vi "Table_GetNodeInformation.vi"(8 "error in (no error)":errorcluster, 9 "TreeBrowser":refnum<k24>, 11 "reference":refnum<k24>) -> (0 "error IO":errorcluster, 3 "Channels":T1[](array[typedef]))   [LabVIEW 2012, in "TableSupportLib.lvlib"]
uses:
  TableSupportLib.lvlib
  NationalInstruments.VeriStand.SystemStorage
  Table_ChannelInfoCluster.ctl
  NationalInstruments.VeriStand.SystemStorageUI
  NationalInstruments.VeriStand.SystemDefinitionAPI
  <vilib>/NI Veristand/Custom Device Offline API/Custom Device Offline API.lvlib
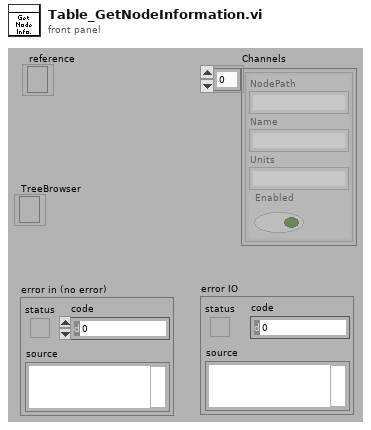
[diagram p1: front panel]
types:
  T1 = typedef "TableSupportLib.lvlib/Table_ChannelInfoCluster.ctl" = cluster{"NodePath":string, "Name":string, "Units":string, "Enabled":bool}
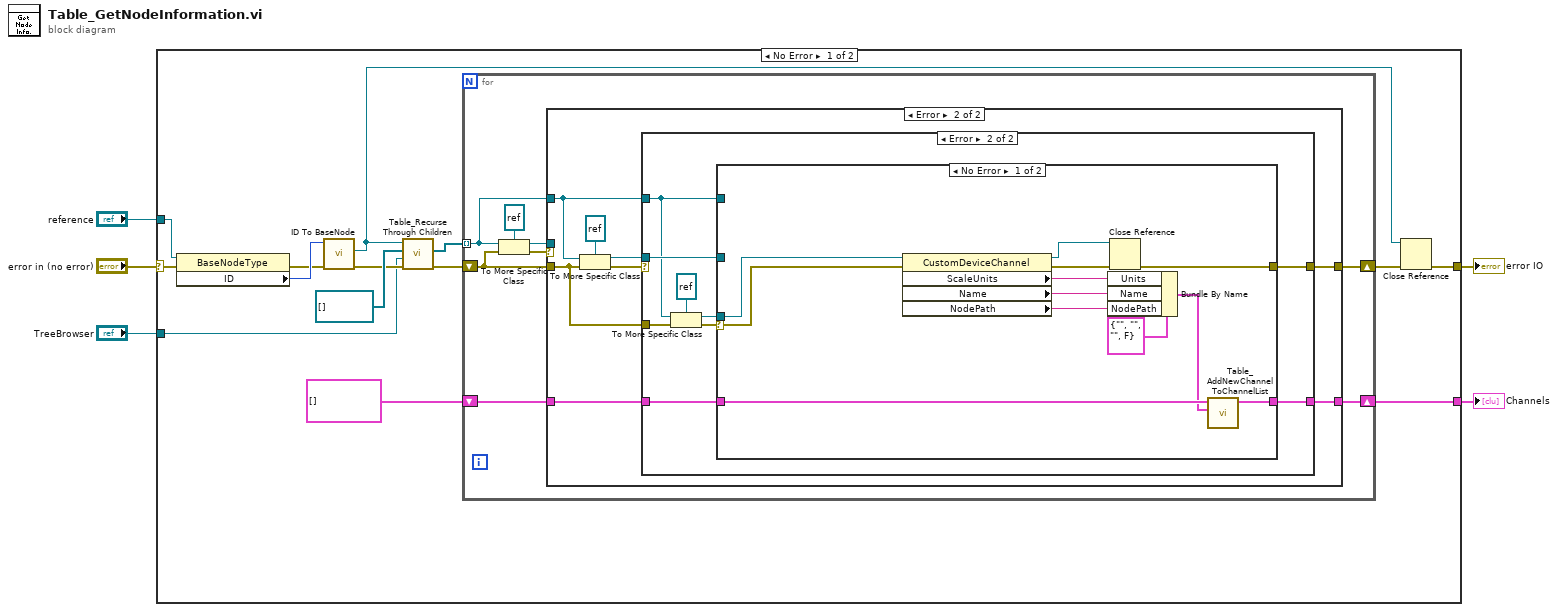
[diagram p0: block diagram]
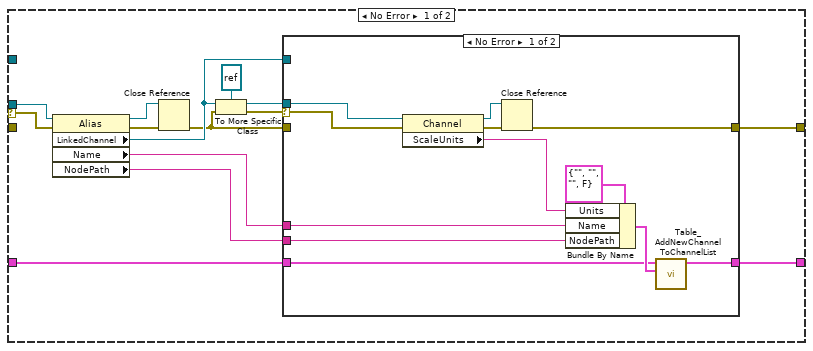
[diagram p2: hidden frame]
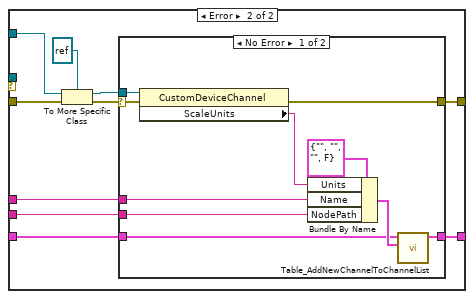
[diagram p3: hidden frame]
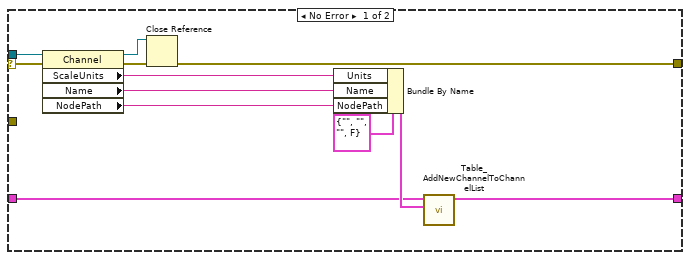
[diagram p5: hidden frame]
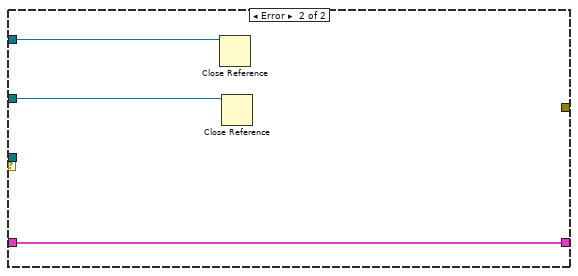
[diagram p6: hidden frame]
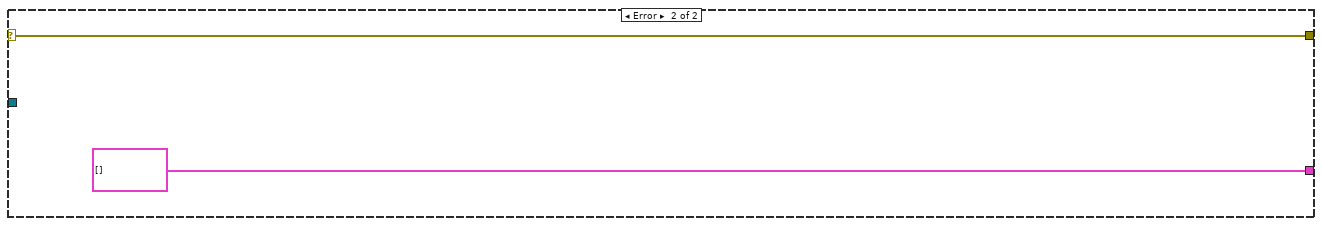
[diagram p7: hidden frame]
diagram:
  n1 = case shown="No Error" "error in (no error)" {
    selector: "error in (no error)" -> [w17 w120]
    tunnel: "reference" -> [w18 _]
    tunnel: [w12 T1[] []] -> w2
    tunnel: [w9 w120] -> w4
    tunnel: "TreeBrowser" -> [w6 _]
    frame No Error {
      n2 = property class="BaseNodeType"(reference=w18, error in=w17) -> (error out=w16:errorcluster, "ID"=w19:u64)  [unwired: 1 out]
      n3 = call <vilib>:"ID To BaseNode.vi"("error in (no error)"=w16, "ID in"=w19) -> ("error out"=w14:errorcluster, "BaseNode"=w7:refnum<k24>)  [unwired: 7 in, 1 out]
      n4 = call "Table_Recurse Through Children.vi"("error in"=w14, "TreeBrowser"=w6, "Children"=refnum<k24>[] [], ".NET Refnum in"=w7) -> ("error out"=w8:errorcluster, "Children"=w11:refnum<k24>[])  [unwired: 6 in]
      n5 = for {
        tunnel: w11 -> [w20] mode=indexing
        shift-right: [w24] -> w12
        shift-left: T1[] [] -> [w23]
        shift-right: [w22] -> w10
        shift-left: w8 -> [w25]
        n6 = To More Specific Class(target class=refnum<k24> refnum ("new reference"), reference=w20, error in=w25) -> (specific class reference=w21:refnum<k24>, error out=w26:errorcluster)
        n7 = case shown="Error" w26 {
          selector: w26 -> [w40 _]
          tunnel: [w34 w82] -> w22
          tunnel: w21 -> [w39 _]
          tunnel: w20 -> [_ w78]
          tunnel: w25 -> [_ w75]
          tunnel: [w35 w77] -> w24
          tunnel: w23 -> [w31 w76]
          frame No Error {
            n8 = property class="Alias"(reference=w39, error in=w40) -> (reference out=w36:refnum<k24>, error out=w37:errorcluster, "LinkedChannel"=w29:refnum<k24>, "Name"=w33:string, "NodePath"=w32:string)
            n9 = Close Reference(reference=w36, error in (no error)=w37) -> (error out=w28:errorcluster)
            n10 = To More Specific Class(target class=refnum<k24> refnum ("new reference"), reference=w29, error in=w28) -> (specific class reference=w38:refnum<k24>, error out=w30:errorcluster)
            n11 = case shown="No Error" w30 {
              selector: w30 -> [w42 _]
              tunnel: w38 -> [w53 _]
              tunnel: [w52 w56] -> w35
              tunnel: [w50 w58] -> w34
              tunnel: w33 -> [w45 w54]
              tunnel: w32 -> [w44 w55]
              tunnel: w31 -> [w43 w57]
              tunnel: w29 -> [_ w63]
              tunnel: w28 -> [_ w62]
              frame No Error {
                n12 = property class="Channel"(reference=w53, error in=w42) -> (reference out=w49:refnum<k24>, error out=w51:errorcluster, "ScaleUnits"=w46:string)
                n13 = Close Reference(reference=w49, error in (no error)=w51) -> (error out=w50:errorcluster)
                n14 = Bundle By Name(cluster=T1 {"NodePath"="", "Name"="", "Units"="", "Enabled"=FALSE}, "Units"=w46, "Name"=w45, "NodePath"=w44) -> (w47:T1)
                n15 = call "Table_AddNewChannelToChannelList.vi"("Channel"=w47, "Channels"=w43) -> ("Channels Out"=w52:T1[])  [unwired: 9 in]
              }
              frame Error {
                n16 = To More Specific Class(target class=refnum<k24> refnum ("new reference"), reference=w63, error in=w62) -> (specific class reference=w60:refnum<k24>, error out=w59:errorcluster)
                n17 = case shown="No Error" w59 {
                  selector: w59 -> [w72 _]
                  tunnel: w60 -> [w73 _]
                  tunnel: [w71 _] -> w58
                  tunnel: w57 -> [w68 w74]
                  tunnel: [w67 w74] -> w56
                  tunnel: w55 -> [w66 _]
                  tunnel: w54 -> [w65 _]
                  frame No Error {
                    n18 = property class="CustomDeviceChannel"(reference=w73, error in=w72) -> (error out=w71:errorcluster, "ScaleUnits"=w64:string)  [unwired: 1 out]
                    n19 = Bundle By Name(cluster=T1 {"NodePath"="", "Name"="", "Units"="", "Enabled"=FALSE}, "Units"=w64, "Name"=w65, "NodePath"=w66) -> (w69:T1)
                    n20 = call "Table_AddNewChannelToChannelList.vi"("Channel"=w69, "Channels"=w68) -> ("Channels Out"=w67:T1[])  [unwired: 9 in]
                  }
                  frame Error {
                  }
                }
              }
            }
          }
          frame Error {
            n21 = To More Specific Class(target class=refnum<k24> refnum ("new reference"), reference=w78, error in=w75) -> (specific class reference=w80:refnum<k24>, error out=w79:errorcluster)
            n22 = case shown="Error" w79 {
              selector: w79 -> [w93 _]
              tunnel: [w90 w95] -> w82
              tunnel: w80 -> [w85 w103]
              tunnel: w78 -> [_ w100]
              tunnel: [w86 w96] -> w77
              tunnel: w76 -> [w87 w97]
              tunnel: w75 -> [_ w101]
              frame No Error {
                n23 = property class="Channel"(reference=w85, error in=w93) -> (reference out=w89:refnum<k24>, error out=w91:errorcluster, "ScaleUnits"=w83:string, "Name"=w94:string, "NodePath"=w84:string)
                n24 = Close Reference(reference=w89, error in (no error)=w91) -> (error out=w90:errorcluster)
                n25 = Bundle By Name(cluster=T1 {"NodePath"="", "Name"="", "Units"="", "Enabled"=FALSE}, "Units"=w83, "Name"=w94, "NodePath"=w84) -> (w88:T1)
                n26 = call "Table_AddNewChannelToChannelList.vi"("Channel"=w88, "Channels"=w87) -> ("Channels Out"=w86:T1[])  [unwired: 9 in]
              }
              frame Error {
                n27 = To More Specific Class(target class=refnum<k24> refnum ("new reference"), reference=w100, error in=w101) -> (specific class reference=w98:refnum<k24>, error out=w99:errorcluster)
                n28 = case shown="No Error" w99 {
                  selector: w99 -> [w115 _]
                  tunnel: w103 -> [_ w118]
                  tunnel: w100 -> [_ w117]
                  tunnel: w98 -> [w114 _]
                  tunnel: w97 -> [w109 w116]
                  tunnel: [w108 w116] -> w96
                  tunnel: [w105 _] -> w95
                  frame No Error {
                    n29 = property class="CustomDeviceChannel"(reference=w114, error in=w115) -> (reference out=w104:refnum<k24>, error out=w106:errorcluster, "ScaleUnits"=w110:string, "Name"=w111:string, "NodePath"=w112:string)
                    n30 = Bundle By Name(cluster=T1 {"NodePath"="", "Name"="", "Units"="", "Enabled"=FALSE}, "Units"=w110, "Name"=w111, "NodePath"=w112) -> (w107:T1)
                    n31 = Close Reference(reference=w104, error in (no error)=w106) -> (error out=w105:errorcluster)
                    n32 = call "Table_AddNewChannelToChannelList.vi"("Channel"=w107, "Channels"=w109) -> ("Channels Out"=w108:T1[])  [unwired: 9 in]
                  }
                  frame Error {
                    n33 = Close Reference(reference=w117) -> ()  [unwired: 1 in, 1 out]
                    n34 = Close Reference(reference=w118) -> ()  [unwired: 1 in, 1 out]
                  }
                }
              }
            }
          }
        }
      }
      n35 = Close Reference(reference=w7, error in (no error)=w10) -> (error out=w9:errorcluster)
    }
    frame Error {
    }
  }
  "error IO" <- w4
  "Channels" <- w2
